vi "Module Init.vi"(8 "error in (no error)":errorcluster, 11 "GUI Helper in":refnum<class "GUI Helper.lvclass">) -> (0 "error out":errorcluster, 3 "GUI Helper out":refnum<class "GUI Helper.lvclass">)   [LabVIEW 2020, in "VolatusGUI.lvlib" / "GUI Helper.lvclass"]
uses:
  GUI Helper.lvclass
  C:/dev/lv20CE/relink/lv-volatus/Volatus/Module/Module.lvclass
  GUI Helper.lvclass/GUI Helper.ctl
  Volatus/Module/Module.lvclass/Module.ctl
  Volatus/MessageQ/MessageQ.lvclass/MessageQ.ctl
  Volatus/Module/Self Q.vi
  Volatus/MessageQ/Send.vi
  Volatus/Module/Module.lvclass
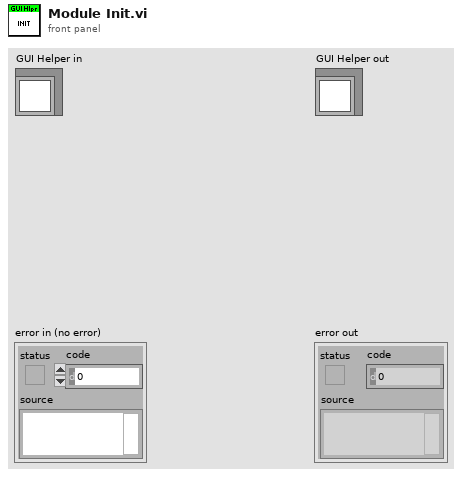
[diagram p1: front panel]
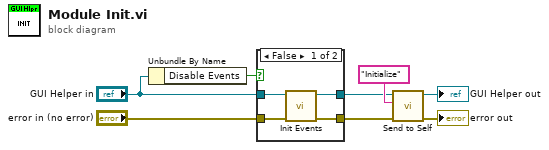
[diagram p0: block diagram]
diagram:
  n1 = Unbundle By Name("GUI Helper in") -> ("Disable Events"=w3:bool)
  n2 = case shown="False" w3 {
    tunnel: "error in (no error)" -> [w12 w13]
    tunnel: [w11 w13] -> w1
    tunnel: [w10 w14] -> w2
    tunnel: "GUI Helper in" -> [w9 w14]
    frame False {
      n3 = call "Init Events.vi"("error in (no error)"=w12, "GUI Helper in"=w9) -> ("error out"=w11:errorcluster, "GUI Helper out"=w10:refnum<class "GUI Helper.lvclass">)  [unwired: 8 in]
    }
    frame True {
    }
  }
  n4 = call "Send to Self.vi"("error in (no error)"=w1, "Message ID"="Initialize", "Module in"=w2) -> ("error out"=→"error out":errorcluster, "Module out"=→"GUI Helper out":refnum<class "GUI Helper.lvclass">)  [unwired: 7 in]
